vi "Darstellung2.vi"(1 "MethodenNamen":string[](array[string])) -> (0 "Darstellung":i8)   [LabVIEW 2010]
uses:
  GVMethode.vi
  GVAbschalten.vi
panel:
  in  "Methode wechseln":bool
  out "derzeitigeMethode":string
  in  "neue Methode":i8(ring) items=["Methode Nr.1", "Methodä Nr.2", "Methadone R3"]
  in  "MethodeVerändern":bool
  in  "Abschalten":bool
  in  "Darstellung":i8(ring) items=["Darstellung1", "Darstellung2", "Darstellung3"]
  in  "Darstellung wechseln":bool
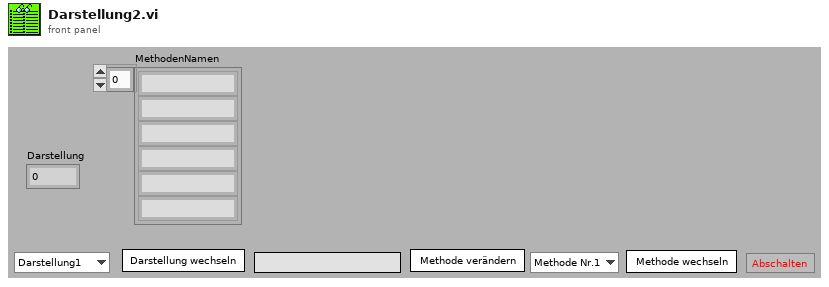
[diagram p1: front panel]
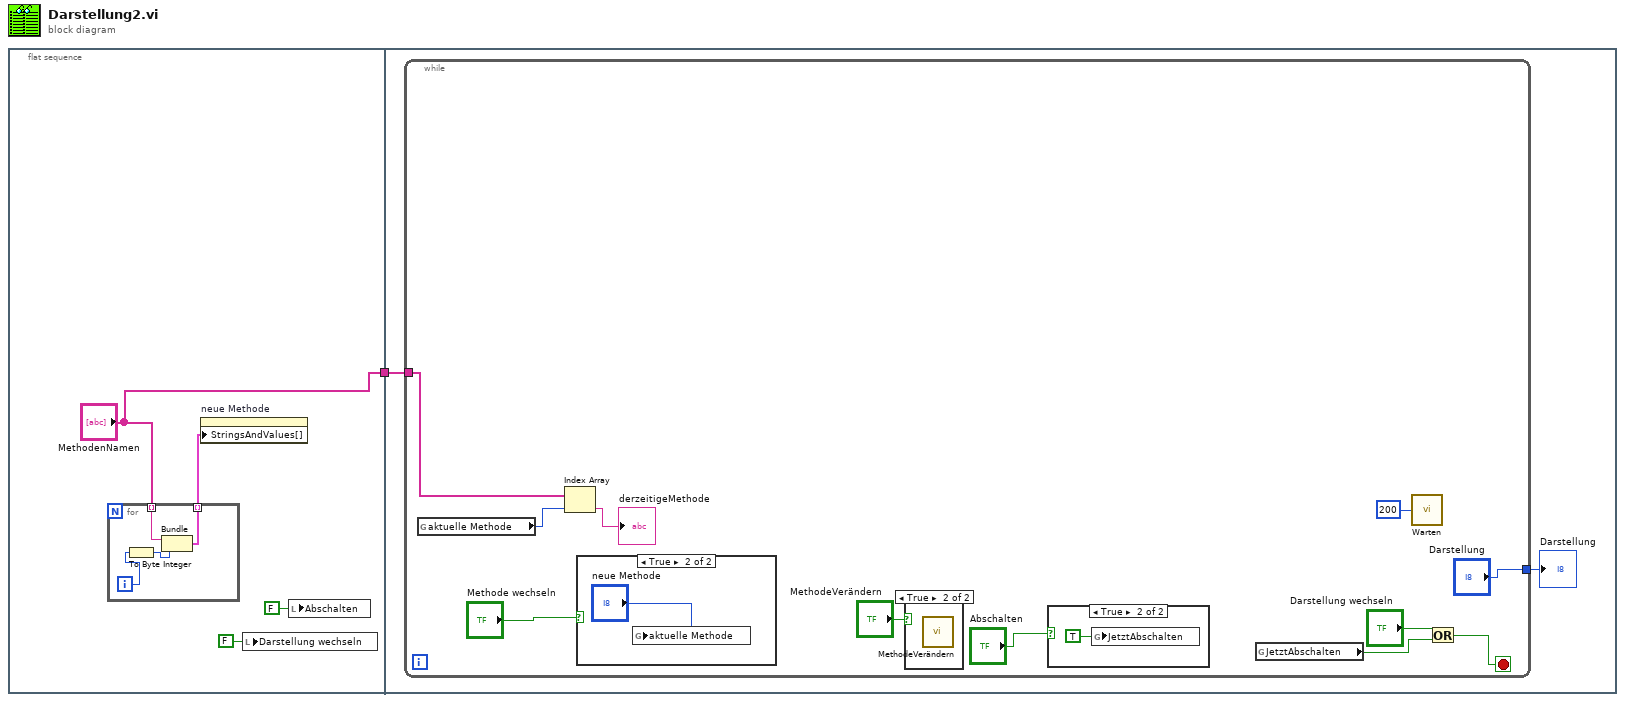
[diagram p0: block diagram]
diagram:
  n1 = flat-sequence {
    tunnel: ["MethodenNamen"] -> w1
    tunnel: w1 -> [w11]
    frame #0 {
      n2 = for {
        tunnel: "MethodenNamen" -> [w9] mode=indexing
        tunnel: [w6] -> w5 mode=indexing
        i -> [w8]
        n3 = To Byte Integer(number=w8) -> (8bit integer=w7:i8)
        n4 = Bundle(w9, w7) -> (w6:cluster{string, i8})  [unwired: 1 in]
      }
      n5 = property on="neue Methode" class="Ring (strikt)"("StringsAndValues[]"=w5) -> ()  [unwired: 2 in, 2 out]
      n6 = local write "Darstellung wechseln"(FALSE ("Darstellung wechseln")) -> ()
      n7 = local write "Abschalten"(FALSE ("Abschalten")) -> ()
    }
    frame #1 {
      n8 = while {
        tunnel: w11 -> [w15]
        tunnel: ["Darstellung"] -> w10
        stop <- w19 stop-if-true
        n9 = global read "GVMethode.vi" "aktuelle Methode"() -> (w14:i8)
        n10 = Index Array(array=w15, index=w14) -> (element=→"derzeitigeMethode":string)
        n11 = case shown="True" "Methode wechseln" {
          frame False {
          }
          frame True {
            n12 = global write "GVMethode.vi" "aktuelle Methode"("neue Methode") -> ()
          }
        }
        n13 = case shown="True" "MethodeVerändern" {
          frame False {
          }
          frame True {
            n14 = call "MethodeVerändern.vi"() -> ()  [unwired: 12 in]
          }
        }
        n15 = case shown="True" "Abschalten" {
          frame False {
          }
          frame True {
            n16 = global write "GVAbschalten.vi" "JetztAbschalten"(TRUE ("JetztAbschalten")) -> ()
          }
        }
        n17 = global read "GVAbschalten.vi" "JetztAbschalten"() -> (w20:bool)
        n18 = call "Warten"("Count(mSec)"=u32 200) -> ()  [unwired: 1 out]
        n19 = Or(x="Darstellung wechseln", y=w20) -> (x .or. y?=w19:bool)
      }
      "Darstellung" <- w10
    }
  }
